vi "HP1200_060_set_CtrlViaInt.vi"(7 "device_addr":u16=22, 8 "error in":errorcluster, 10 "CtrlViaInt_in":u8=2, 11 "conn_id_in":refnum<k5>) -> (0 "error out":errorcluster, 1 "response":string, 2 "CtrlViaInt":u8, 3 "conn_id_out":refnum<k5>, 4 "status":bool)   [LabVIEW 2019]
panel:
  # "1 = Remote\n2 = RS-485\n255 = Unlock"
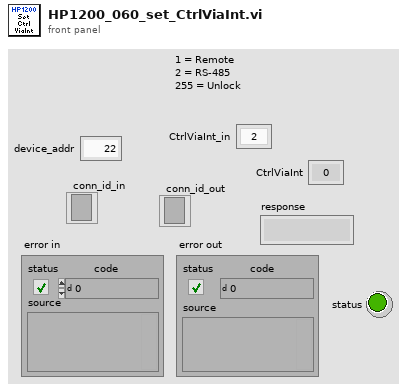
[diagram p1: front panel]
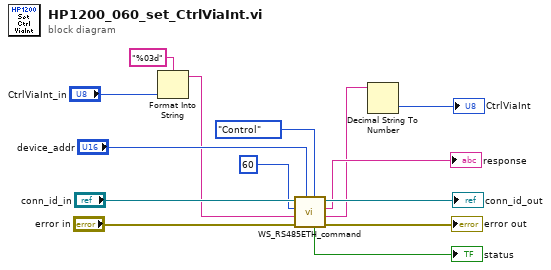
[diagram p0: block diagram]
diagram:
  n1 = Format Into String(format string="%03d", "CtrlViaInt_in") -> (resulting string=w1:string)  [unwired: 2 in, 1 out]
  n2 = call "WS_RS485ETH_command.vi"("action"=enum16{"Request", "Control"}."Control", "device_addr"="device_addr", "error in"="error in", "data_string"=w1, "param_num"=u16 60, "conn_id_in"="conn_id_in") -> ("error out"=→"error out":errorcluster, "data_out"=w5:string, "response"=→"response":string, "conn_id_out"=→"conn_id_out":refnum<k5>, "status"=→"status":bool)  [unwired: 1 in]
  n3 = Decimal String To Number(string=w5) -> (number=→"CtrlViaInt":i32)  [unwired: 2 in, 1 out]
